vi "CheckReplace.vi"(10 "DisabledEnum":T1(ring)) -> (2 "Replace?":bool)   [LabVIEW 2022 SP3]
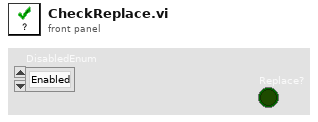
[diagram p1: front panel]
types:
  T1 = enum8{"Enabled", "Disabled", "Disabled and Grayed Out"}
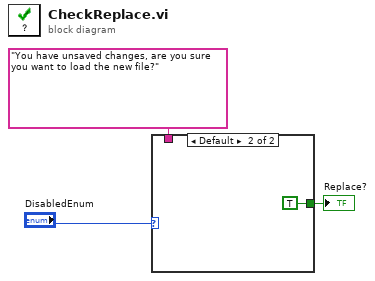
[diagram p0: block diagram]
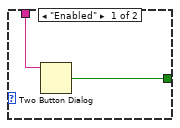
[diagram p2: hidden frame]
diagram:
  n1 = case shown="Default" "DisabledEnum" {
    tunnel: "You have unsaved changes, are you sure you want to load the new file?" ("message") -> [w5 _]
    tunnel: [w4 TRUE ("T button?")] -> w1
    frame "Enabled" {
      n2 = Two Button Dialog(message=w5) -> (T button?=w4:bool)  [unwired: 2 in]
    }
    frame Default {
    }
  }
  "Replace?" <- w1
